vi "Make Color String.vi"(7 "Prefix (color:0x)":string="color:0x", 8 "error in (no error)":errorcluster, 9 "Opacity (255)":u8=255, 10 "Color":u32) -> (0 "error out":errorcluster, 2 "color string":string)   [LabVIEW 2012]
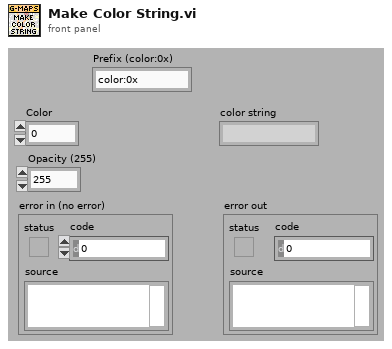
[diagram p1: front panel]
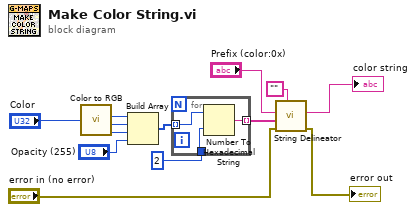
[diagram p0: block diagram]
diagram:
  n1 = call <vilib>:"Color to RGB.vi"("Color"="Color") -> ("R"=w3:u8, "G"=w4:u8, "B"=w5:u8)  [unwired: 1 out]
  n2 = Build Array(w3, w4, w5, "Opacity (255)") -> (w6:u8[])
  n3 = for {
    tunnel: w6 -> [w16] mode=indexing
    tunnel: i16 2 ("width (-)") -> [w15]
    tunnel: [w14] -> w8 mode=indexing
    n4 = Number To Hexadecimal String(1:w15, 2:w16) -> (0:w14:string)
  }
  n5 = call "String Delineator.vi"("Delineator \"&\""="", "error in (no error)"="error in (no error)", "Array of Strings"=w8, "Base String"="Prefix (color:0x)") -> ("error in (no error)"=→"error out":errorcluster, "New String"=→"color string":string)  [unwired: 6 in]
